vi "ExFileReadNDisplayRGBGainOffsetTif.vi"() -> ()   [LabVIEW 2010]
panel:
  in  "TIF output":path=path "C:/Program Files/SIToolKit/LabVIEW/Data Files/test"
  out "Blue Offset":dbl format="%.2f"
  out "Green Offset":dbl format="%.2f"
  out "Red Offset":dbl format="%.2f"
  out "Blue Gain":dbl format="%.2f"
  out "Green Gain":dbl format="%.2f"
  out "Red Gain":dbl format="%.2f"
  in  "Blue Offset":dbl format="%.2f"
  in  "Green Offset":dbl format="%.2f"
  in  "Red Offset":dbl format="%.2f"
  in  "Blue Gain":dbl=1.0 format="%.2f"
  in  "Red Gain":dbl=1.0 format="%.2f"
  in  "Green Gain":dbl=1.0 format="%.2f"
  in  "Bit shift":u16
  in  "Type of Bayer":u32=1 max=4 step=1
  in  "Full File Name":path=path "C:/Program Files/SIToolKit/LabVIEW/Data Files/Color.SPE"
  in  "?":bool
  in  "FileType":u32=67371008
  out "error out":errorcluster
  in  "error in (no error)":errorcluster
  # "ExReadFileNDisplayRGBGainOffsetTif.vi\nThis example will read in a file of the selected data type and display as RGB frame. This example also sets the gain and offset to be applied to each color\nin the Bayer pattern. When finished viewing data, make sure to use the STOP button to close the display."
  # "File Types:\nSPE = 67371008\nTIF   = 67174400\nPMI  = 67436544"
  # "This will properly close\nthe image and\ndeallocate memory."
  # "Browse match pattern is set to *.spe.  Modify this if different file type is needed."
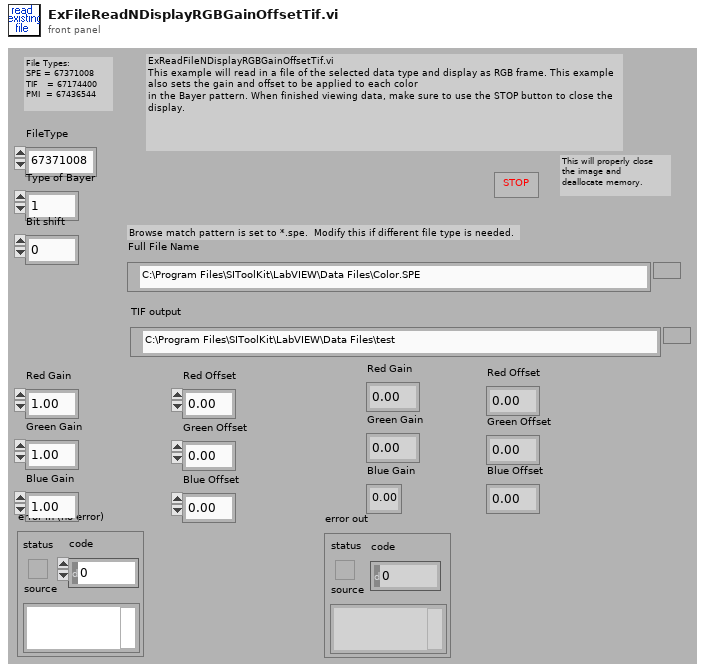
[diagram p1: front panel]
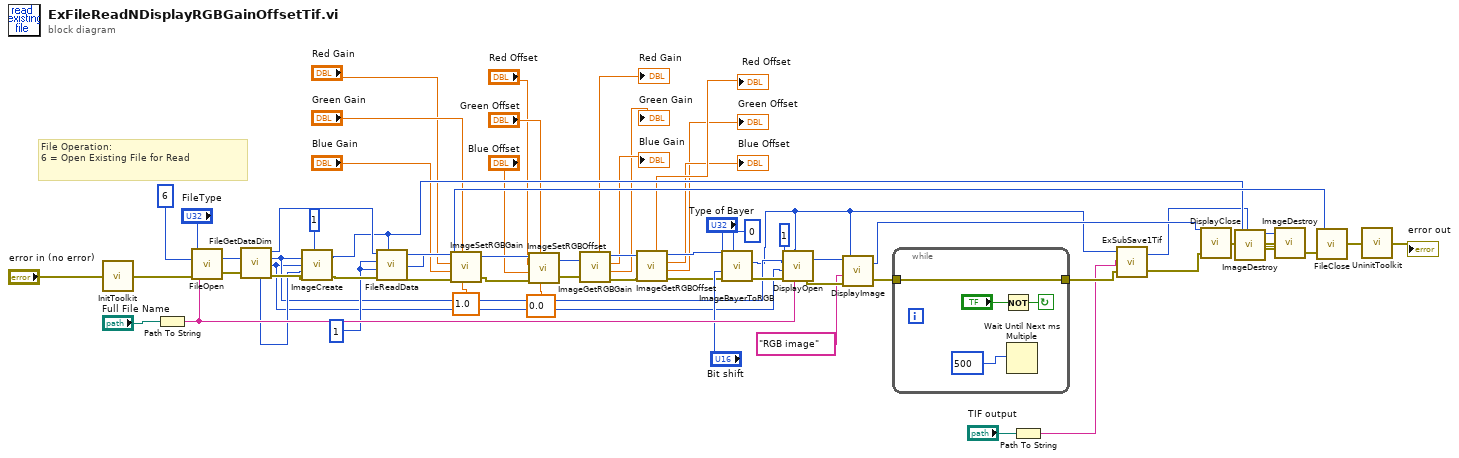
[diagram p0: block diagram]
diagram:
  w45 = 1
  # "File Operation:\n6 = Open Existing File for Read"
  n1 = call <userlib>:"InitToolkit.vi"("error in"="error in (no error)") -> ("error out"=w61:errorcluster)
  n2 = Path To String(path="Full File Name") -> (string=w50:string)
  n3 = call <userlib>:"FileOpen.vi"("error in"=w61, "File Operations"=u32 6 ("File Operation"), "FileName"=w50, "File Type"="FileType") -> ("error out"=w59:errorcluster, "File Handle"=w58:u32)
  n4 = call <userlib>:"FileGetDataDim.vi"("File Handle"=w58, "error in"=w59) -> ("Data Type"=w35:u32, "File Handle"=w47:u32, "X dim"=w9:u32, "Y dim"=w8:u32, "error out"=w57:errorcluster)  [unwired: 1 out]
  n5 = call <userlib>:"ImageCreate.vi"("X dimension"=w9, "Y dimension"=w8, "Data Type"=w35, "error in"=w57, "Number Of Frames"=1) -> ("Image Handle"=w37:u32, "error out"=w46:errorcluster)
  n6 = call <userlib>:"FileReadData.vi"("File Handle"=w47, "Start Frame"=w45, "End Frame"=w45, "error in"=w46, "Image Handle"=w37) -> ("File Handle"=w44:u32, "Image Handle"=w33:u32, "error out"=w32:errorcluster)
  n7 = call <userlib>:"ImageSetRGBGain.vi"("reserved"=1.0, "Green Gain"="Green Gain", "error in (no error)"=w32, "Blue Gain"="Blue Gain", "Red Gain"="Red Gain", "Image Handle"=w33) -> ("error out"=w30:errorcluster, "Image Handle"=w31:u32)
  n8 = call <userlib>:"ImageSetRGBOffset.vi"("reserved"=0.0, "Green Offset"="Green Offset", "error in (no error)"=w30, "Blue Offset"="Blue Offset", "Red Offset"="Red Offset", "Image Handle"=w31) -> ("error out"=w21:errorcluster, "Image Handle"=w16:u32)
  n9 = call <userlib>:"ImageGetRGBGain.vi"("Image Handle"=w16, "error in (no error)"=w21) -> ("Red"=→"Red Gain":dbl, "Image Handle"=w17:u32, "Blue"=→"Blue Gain":dbl, "Green"=→"Green Gain":dbl, "error out"=w20:errorcluster)  [unwired: 1 out]
  n10 = call <userlib>:"ImageGetRGBOffset.vi"("Image Handle"=w17, "error in (no error)"=w20) -> ("Red"=→"Red Offset":dbl, "Image Handle"=w18:u32, "Blue"=→"Blue Offset":dbl, "Green"=→"Green Offset":dbl, "error out"=w19:errorcluster)  [unwired: 1 out]
  n11 = call <userlib>:"ImageBayerToRGB.vi"("Image Handle"=w18, "Type of Bayer"="Type of Bayer", "Shift amount"="Bit shift", "error in"=w19, "RGB Handle In"=0) -> ("RGB Image Handle"=w5:u32, "error out"=w49:errorcluster)  [unwired: 1 out]
  n12 = call <userlib>:"DisplayOpen.vi"("Display Title"=w50, "Image Handle"=w5, "error in"=w49, "Display Height"=w8, "Display Width"=w9, "Display Type"=1) -> ("error out"=w43:errorcluster, "Display Handle"=w42:u32)
  n13 = call <userlib>:"DisplayImage.vi"("error in"=w43, "Title"="RGB image", "Image Handle"=w5, "Display Handle"=w42) -> ("error out"=w36:errorcluster, "Display Handle"=w41:u32)
  n14 = while {
    tunnel: w36 -> [w64]
    tunnel: [w64] -> w7
    stop <- w66 continue-if-true
    n15 = Not(x="?") -> (.not. x?=w66:bool)
    n16 = Wait Until Next ms Multiple(millisecond multiple=500) -> ()  [unwired: 1 out]
  }
  n17 = Path To String(path="TIF output") -> (string=w2:string)
  n18 = call "ExSubSave1Tif.vi"("error in (no error)"=w7, "File name"=w2, "Image Handle"=w5) -> ("error out"=w6:errorcluster, "Image handle"=w4:u32)
  n19 = call <userlib>:"DisplayClose.vi"("error in"=w6, "Display Handle"=w41) -> ("error out"=w54:errorcluster)
  n20 = call <userlib>:"ImageDestroy.vi"("error in"=w54, "Data handle"=w4) -> ("error out"=w40:errorcluster)
  n21 = call <userlib>:"ImageDestroy.vi"("error in"=w40, "Data handle"=w37) -> ("error out"=w39:errorcluster)
  n22 = call <userlib>:"FileClose.vi"("error in"=w39, "File Handle"=w44) -> ("error out"=w53:errorcluster)
  n23 = call <userlib>:"UninitToolkit.vi"("error in"=w53) -> ("error out"=→"error out":errorcluster)
